vi "Integer Check by Formal.vi"(10 "Sudoku Formal In":T1, 11 "Sudoku Int In":u8[][](array[numeric])) -> (2 "Is Modify":bool, 3 "Sudoku Int Out":u8[][](array[numeric]))   [LabVIEW 2015, in "Sudoku Library.lvlib"]
doc: "Created IvanLis by LabVIEW Portal\nProfile: http://labviewportal.org/memberlist.php?mode=viewprofile&u=987\neMail: IvanLisanov@gMail.com\nTelegram: https://t.me/IvanLis"
uses:
  Sudoku Library.lvlib
  TypeDef/Sudoku Formal.ctl
  TypeDef/Cell Formal.ctl
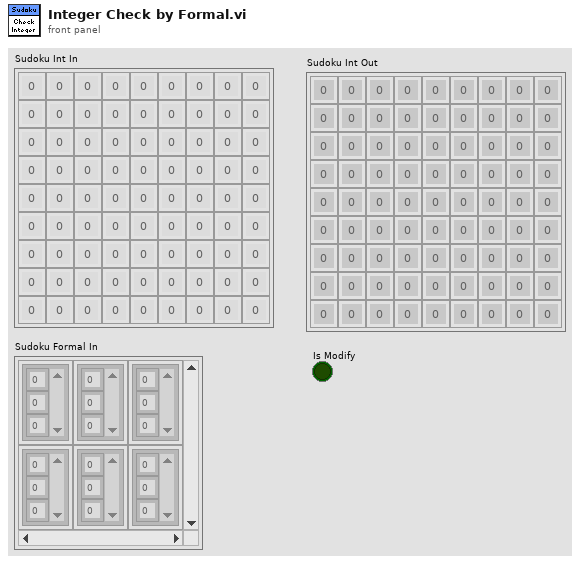
[diagram p1: front panel]
types:
  T1 = typedef "Sudoku Library.lvlib/Sudoku Formal.ctl" = T2[][]
  T2 = typedef "Sudoku Library.lvlib/Cell Formal.ctl" = cluster{"Variant":u8[]}
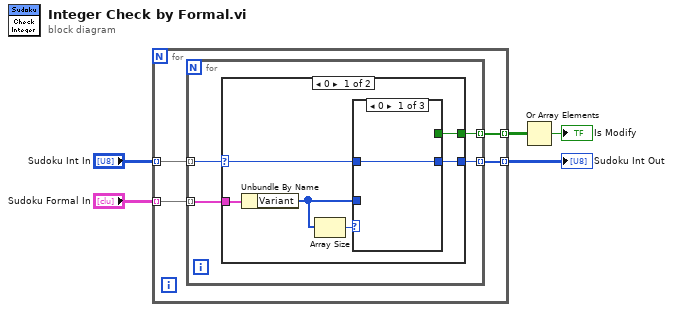
[diagram p0: block diagram]
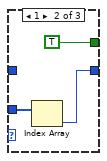
[diagram p2: hidden frame]
diagram:
  n1 = for {
    tunnel: "Sudoku Int In" -> [w9] mode=indexing
    tunnel: "Sudoku Formal In" -> [w8] mode=indexing
    tunnel: [w7] -> w2 mode=indexing
    tunnel: [w6] -> w1 mode=indexing
    n2 = for {
      tunnel: w9 -> [w13] mode=indexing
      tunnel: w8 -> [w12] mode=indexing
      tunnel: [w11] -> w7 mode=indexing
      tunnel: [w10] -> w6 mode=indexing
      n3 = case shown="0" w13 {
        selector: w13 -> [w17 w25]
        tunnel: w12 -> [w19 _]
        tunnel: [w16 w25] -> w11
        tunnel: [w14 _] -> w10
        frame 0 {
          n4 = Unbundle By Name(w19) -> ("Variant"=w15:u8[])
          n5 = Array Size(array=w15) -> (size(s)=w18:i32)
          n6 = case shown="0" w18 {
            tunnel: w17 -> [w20 _ w24]
            tunnel: [w20 w22 w24] -> w16
            tunnel: w15 -> [_ w23 _]
            tunnel: [_ TRUE _] -> w14
            frame 0 {
            }
            frame 1 {
              n7 = Index Array(array=w23) -> (element=w22:u8)  [unwired: 1 in]
            }
            frame 2, Default {
            }
          }
        }
        frame 1, Default {
        }
      }
    }
  }
  "Sudoku Int Out" <- w2
  n8 = Or Array Elements(Boolean array=w1) -> (logical OR=→"Is Modify":bool)
